vi "2'scomplementPGAconv.vi"(4 "Normalize Data":bool=TRUE, 6 "VREF Ratio":dbl=1.0 format="%.04f", 7 "Units":enum16{"Volts", "LSB"}(ring) caption="Units (Volts)", 8 "RefVoltage":dbl=2.4, 9 "Bits":i32=24, 10 "GAIN#":enum16{"1", "2", "4", "6", "8", "12", "24"}(ring) caption="PGA Gain", 11 "Data In":i32[](array[numeric])) -> (3 "Data Out":dbl[](array[numeric]))   [LabVIEW 2010]
doc: "This VI converts the ADC data to the correct units (volts orLSB). It also can scale the data to be input-referred (normalized) or ADC output.\n\nInputs:\n\nData In - (I32[]) ADC data\nPGA Gain - (enum) gain setting of ADC PGA\nUnits - (enum) desired output data units (volts or codes)\nBits - (I32) number of data bits per code\nRefVoltage - (DBL) reference voltage of ADC (used to calculate LSB step size)\nNormalize Data - (boolean) TRUE=input referred data, FALSE=ADC data\n\nOutputs:\nData Out - (DBL[]) data output"
uses:
  Controls/Register/TYP_Reg_CHxSET.ctl
panel:
  in  "CH1SET":T1={"PD#"=enum."Normal Operation", "GAIN#"=enum."6", "SRB2"=enum."Open (Off)", "MUX#"=enum."Normal Electrode"}
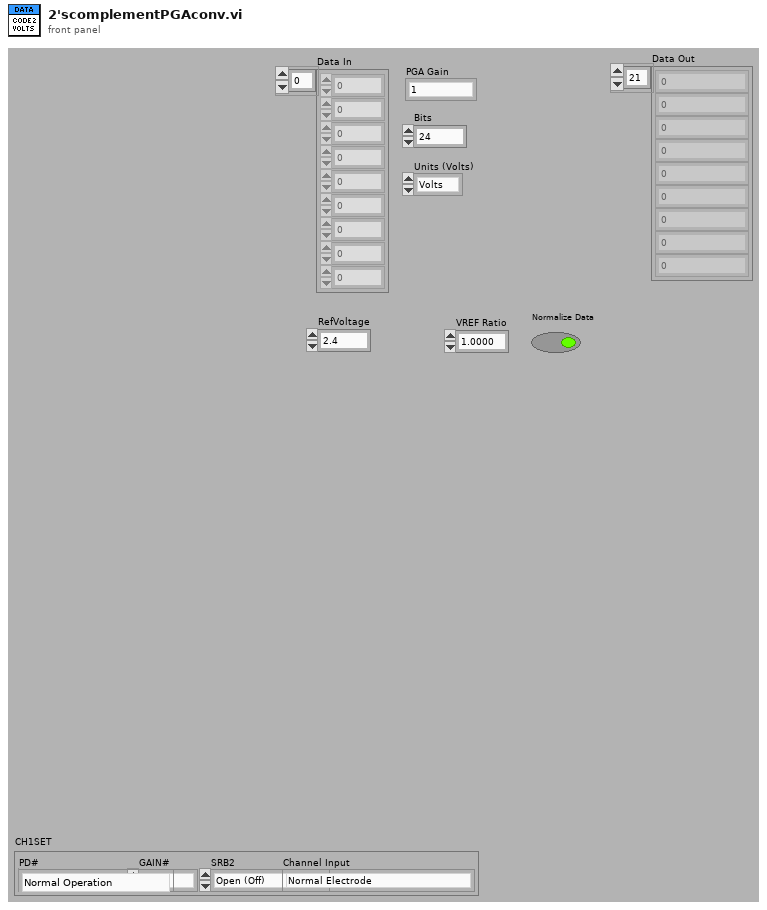
[diagram p1: front panel]
types:
  T1 = typedef "TYP_Reg_CHxSET.ctl" = cluster{"PD#":enum16{"Normal Operation", "Power-down"}, "GAIN#":enum16{"1", "2", "4", "6", "8", "12", "24"}, "SRB2":enum16{"Open (Off)", "Closed (On)"}, "MUX#":enum16{"Normal Electrode", "Input Short", "BIAS Measurement", "MVDD", "Temperature Sensor", "Test Signal", "BIAS Positive Electrode Driver", "BIAS Negative Electrode Driver"}}
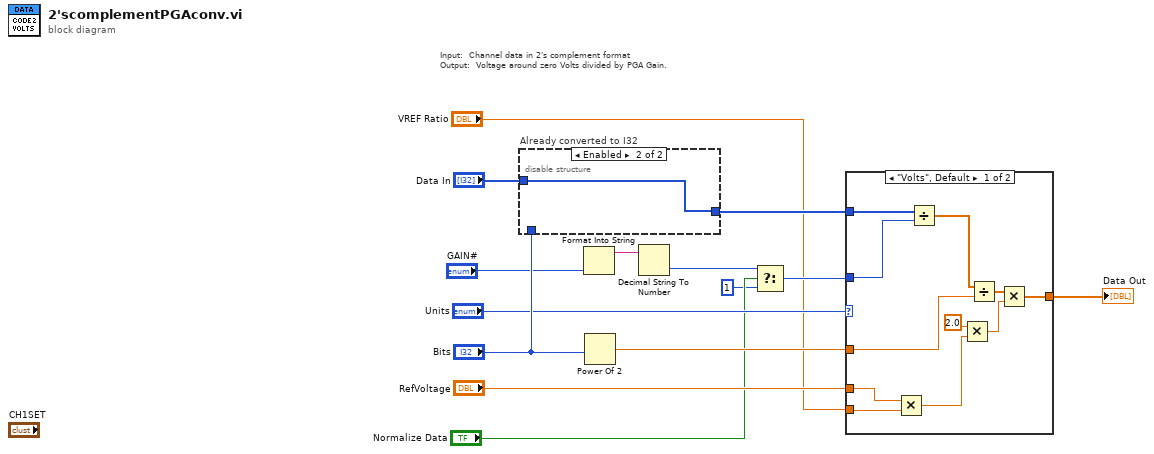
[diagram p0: block diagram]
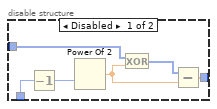
[diagram p2: hidden frame]
diagram:
  # "Input:  Channel data in 2's complement format\nOutput:  Voltage around zero Volts divided by PGA Gain."
  n1 = disable-structure "Already converted to I32" shown="Enabled" {
    disable-tunnel: [w20 w21] -> w13
    disable-tunnel: "Bits" -> [w17 _]
    disable-tunnel: "Data In" -> [w15 w21]
    frame Disabled {
      n2 = Decrement(x=w17) -> (x-1=w18:i32)
      n3 = Power Of 2(x=w18) -> (2^x=w16:dbl)
      n4 = Exclusive Or(1:w16, 2:w15) -> (0:w19:i32[])
      n5 = Subtract(x=w19, y=w16) -> (x-y=w20:dbl[])
    }
    frame Enabled {
    }
  }
  n6 = Format Into String("GAIN#") -> (resulting string=w8:string)  [unwired: 3 in, 1 out]
  n7 = Power Of 2(x="Bits") -> (2^x=w14:dbl)
  n8 = Decimal String To Number(string=w8) -> (number=w6:i32)  [unwired: 3 out]
  n9 = Select(t=w6, s="Normalize Data", f=1) -> (s? t:f=w5:i32)
  n10 = case shown="\"Volts\", Default" "Units" {
    tunnel: w14 -> [w32 _]
    tunnel: w13 -> [w31 w33]
    tunnel: "RefVoltage" -> [w23 _]
    tunnel: [w26 w33] -> w11
    tunnel: w5 -> [w25 _]
    tunnel: "VREF Ratio" -> [w24 _]
    frame "Volts", Default {
      n11 = Multiply(x=w23, y=w24) -> (x*y=w22:dbl)
      n12 = Divide(x=w31, y=w25) -> (x/y=w30:dbl[])
      n13 = Multiply(x=2.0, y=w22) -> (x*y=w27:dbl)
      n14 = Divide(x=w30, y=w32) -> (x/y=w28:dbl[])
      n15 = Multiply(x=w28, y=w27) -> (x*y=w26:dbl[])
    }
    frame "LSB" {
    }
  }
  "Data Out" <- w11
